vi "GetWindowPosition.vi"(8 "No Error":errorcluster, 11 "Window [SDL_Window *]":T1 format="%.0x") -> (0 "Error Out":errorcluster, 2 "y":i32, 3 "x":i32)   [LabVIEW 2026, in "SDL3.lvlib" / "Video.lvlib"]
doc: "<B>Summary</B>\nGet the position of a window.\n\n<B>Remarks</B>\nThis is the current position of the window as last reported by the windowing system."
uses:
  Video.lvlib
  <vilib>/Utility/error.llb/Error Cluster From Error Code.vi
  Error/Error.lvlib
  Lib/SDL3.dll
  SDL_Window--pointer.ctl
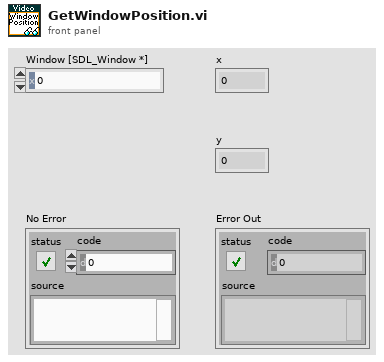
[diagram p1: front panel]
types:
  T1 = typedef "SDL3.lvlib/Video.lvlib/SDL_Window--pointer.ctl" = i64
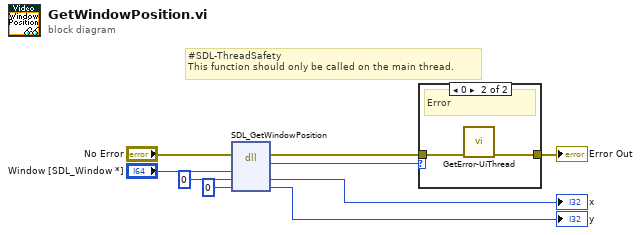
[diagram p0: block diagram]
diagram:
  # "#SDL-ThreadSafety\nThis function should only be called on the main thread."
  n1 = dll-call lib="C:/Users/saukko/Dev/LV-SDL3/Sources/SDL3/Lib/SDL3.*" fn="SDL_GetWindowPosition"(error in="No Error", "window"="Window [SDL_Window *]", "w"=0, "h"=0) -> (error out=w6:errorcluster, "return type"=w5:i32, "w"=→"x":i32, "h"=→"y":i32)  [unwired: 3 in, 1 out]
  n2 = case shown="0" w5 {
    tunnel: w6 -> [w10 w12]
    tunnel: [w10 w11] -> w8
    frame Default {
      # "Ok"
    }
    frame 0 {
      # "Error"
      n3 = call "GetError-UiThread.vi"("No Error"=w12) -> ("error out"=w11:errorcluster)  [unwired: 10 in]
    }
  }
  "Error Out" <- w8
